vi "CANOpen Build xPDO DVR.vi"(8 "error in (no error)":errorcluster, 10 "Values Array":dbl[](array[numeric]), 11 "Lookup Table":variant) -> (0 "error out":errorcluster, 3 "xPDO DVR":refnum<data-value>)   [LabVIEW 2011, in "CANOpen Addon Custom Device.lvlib"]
uses:
  CANOpen Addon Custom Device.lvlib
  xPDO DVR.ctl
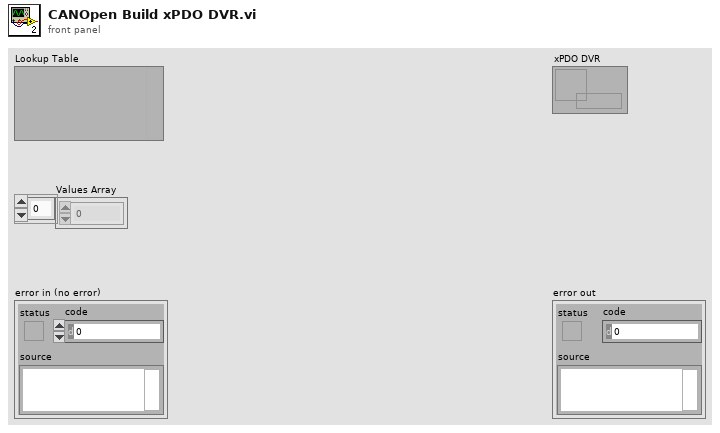
[diagram p1: front panel]
types:
  T1 = typedef "CANOpen Addon Custom Device.lvlib/xPDO DVR.ctl" = cluster{"Lookup Table":variant, "Values Array":dbl[]}
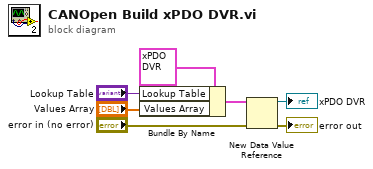
[diagram p0: block diagram]
diagram:
  n1 = Bundle By Name(cluster=T1 {"Lookup Table"=variant, "Values Array"=[]} ("xPDO DVR"), "Lookup Table"="Lookup Table", "Values Array"="Values Array") -> (w4:T1)
  n2 = New Data Value Reference(data value=w4, error in="error in (no error)") -> (data value reference=→"xPDO DVR":refnum<data-value>, error out=→"error out":errorcluster)
